vi "ConvertHeaterStateToDisplay.vi"(11 "Standby?":bool) -> (3 "Heater Display State":T1)   [LabVIEW 2012]
uses:
  HeaterDisplayState.ctl
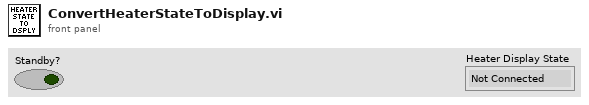
[diagram p1: front panel]
types:
  T1 = typedef "HeaterDisplayState.ctl" = enum16{"Not Connected", "Run", "Standby"}
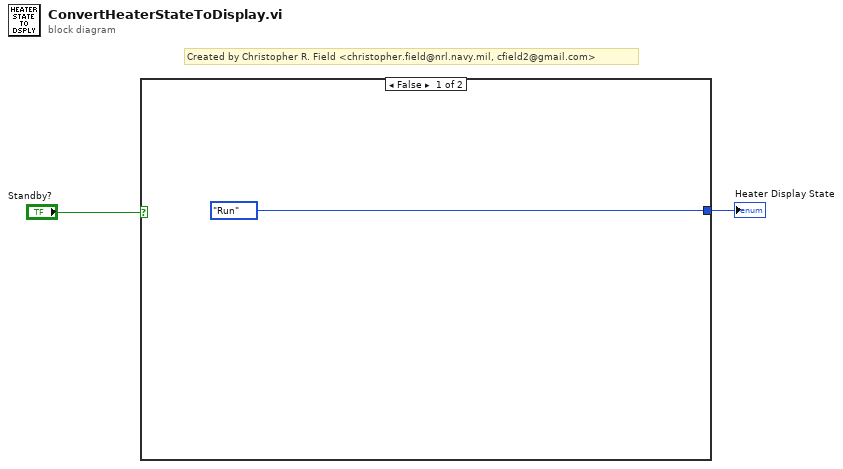
[diagram p0: block diagram]
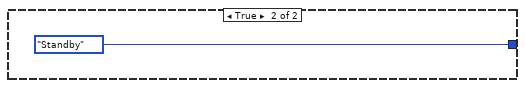
[diagram p2: hidden frame]
diagram:
  # "Created by Christopher R. Field <christopher.field@nrl.navy.mil, cfield2@gmail.com>"
  n1 = case shown="False" "Standby?" {
    tunnel: [HeaterDisplayState."Run" ("Heater Display State") HeaterDisplayState."Standby" ("Heater Display State")] -> w2
    frame False {
    }
    frame True {
    }
  }
  "Heater Display State" <- w2
